vi "Set-options.vi"(8 "error in (no error)":errorcluster, 10 "Options":T1, 11 "Object ref in":T2) -> (0 "error out":errorcluster, 3 "Object ref out":T2)   [LabVIEW 2013, in "MaterialCharacterization.lvlib" / "MC-Main.lvclass"]
uses:
  MC-Main.lvclass
  Object-reference.ctl
  Options.ctl
  MC-Main.lvclass/MC-Main.ctl
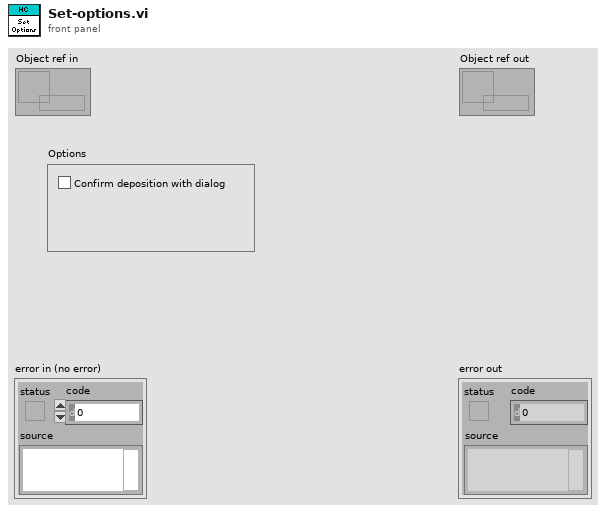
[diagram p1: front panel]
types:
  T1 = typedef "MaterialCharacterization.lvlib/MC-Main.lvclass/Options.ctl" = cluster{"Option 1":bool}
  T2 = typedef "MaterialCharacterization.lvlib/MC-Main.lvclass/Object-reference.ctl" = refnum<data-value>
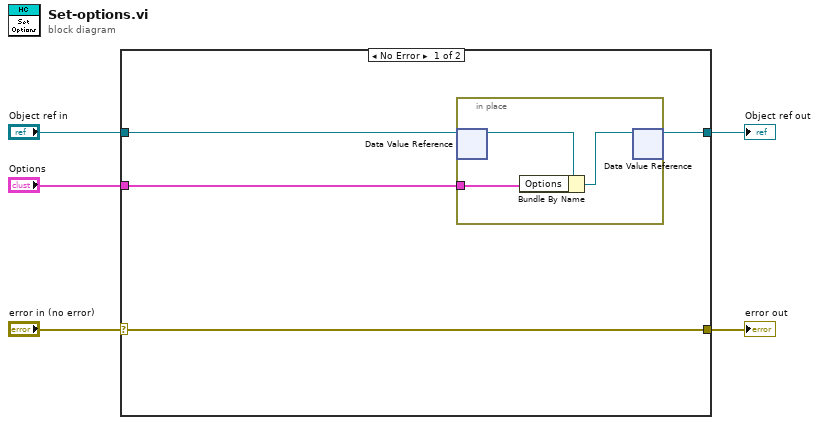
[diagram p0: block diagram]
diagram:
  n1 = case shown="No Error" "error in (no error)" {
    selector: "error in (no error)" -> [w9 w14]
    tunnel: [w9 w14] -> w4
    tunnel: [w7 w13] -> w2
    tunnel: "Object ref in" -> [w8 w13]
    tunnel: "Options" -> [w6 _]
    frame No Error {
      n2 = in-place {
        in-place-border: w6 -> [w12]
        n3 = in-place-dvr #1(w8) -> (w11:refnum<class "MC-Main.lvclass">)  [unwired: 1 out]
        n4 = Bundle By Name(cluster=w11, "Options"=w12) -> (w10:refnum<class "MC-Main.lvclass">)
        n5 = in-place-dvr #1(w10) -> (w7:T2)  [unwired: 1 out]
      }
    }
    frame Error {
    }
  }
  "error out" <- w4
  "Object ref out" <- w2
